vi "Client_next.vi"(10 "lambda":dbl=0.1 format="%#_13g", 11 "Time of previous":dbl) -> (3 "Client":T1)   [LabVIEW 2014, in "LukiBrary.lvlib"]
doc: "Otrzymuje czas poprzedniego klienta, parametr lambda (oczekiwaną liczbę klientów na jednostkę czasu [SEK]). Losuje (tworzy) klienta którego Price wacha się w przedziale (0;50)"
uses:
  LukiBrary.lvlib
  Client.ctl
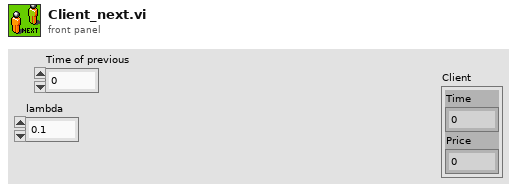
[diagram p1: front panel]
types:
  T1 = typedef "LukiBrary.lvlib/Client.ctl" = cluster{"Time":i32, "Price":i32}
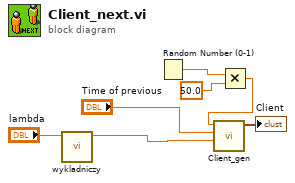
[diagram p0: block diagram]
diagram:
  n1 = call "wykladniczy.vi"("lambda"="lambda") -> ("X~wykładniczy"=w4:dbl)  [unwired: 10 in]
  n2 = Random Number (0-1)() -> (number: 0 to 1=w2:dbl)
  n3 = Multiply(x=w2, y=50.0) -> (x*y=w1:dbl)
  n4 = call "Client_gen.vi"("Różnica"=w4, "Time"="Time of previous", "Price"=w1) -> ("Client"=→"Client":T1)  [unwired: 8 in]
